vi "求最大公约数.vi"(8 "n":i32, 11 "m":i32) -> (3 "gcd(m,n)":i32)   [LabVIEW 2012]
doc: "功能：\n\n利用辗转相除法求整数m、n的最大公约数。\n\nCSXCS_366创建。"
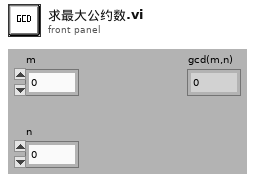
[diagram p1: front panel]
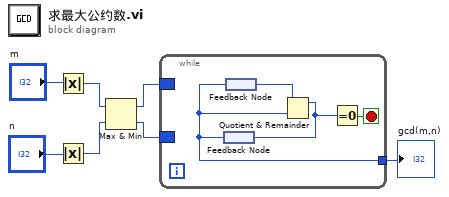
[diagram p0: block diagram]
diagram:
  n1 = Absolute Value(x="m") -> (abs(x)=w5:i32)
  n2 = Absolute Value(x="n") -> (abs(x)=w4:i32)
  n3 = Max & Min(x=w5, y=w4) -> (max(x,y)=w3:i32, min(x,y)=w2:i32)
  n4 = while {
    border: w3 -> [_]
    border: w2 -> [_]
    tunnel: [w8] -> w1
    stop <- w9 stop-if-true
    n5 = feedback #1() -> (w8:i32)
    n6 = feedback-in #2(w8) -> ()
    n7 = feedback #2() -> (w11:i32)
    n8 = Quotient & Remainder(x=w11, y=w8) -> (x-y*floor(x/y)=w10:i32)  [unwired: 1 out]
    n9 = feedback-in #1(w10) -> ()
    n10 = Equal To 0?(x=w10) -> (x = 0?=w9:bool)
  }
  "gcd(m,n)" <- w1
